vi "4461 - Create Reference Waveforms.vi"(8 "error in (no error)":errorcluster, 10 "reset signal":bool, 11 "Lockin.DAQ in":refnum<class "Lockin.DAQ.lvclass">) -> (0 "error out":errorcluster, 2 "Ref Array":waveform(dbl)[](array[waveform]), 3 "Lockin.DAQ out":refnum<class "Lockin.DAQ.lvclass">)   [LabVIEW 2016, in "Lockin.DAQ.lvclass"]
uses:
  Lockin.DAQ.lvclass
  Typedefs/REF-cluster.ctl
  Instrument.Lockinl.UI/Typedefs/REF Channel--Cluster.ctl
  Typedefs/Sampling.ctl
  <vilib>/measure/NI_MABase.lvlib
  Instrument.Lockinl.UI/Instrument.Lockin.UI.lvclass
panel:
  in  "Configuration.Channels: REF":T1 {"Order" min=1; "TC" min=0.0001 format="%#_3p"; "Phase" format="%.3g"; "Frequency" min=0.0001 max=10000.0 format="%.3g"}
  in  "Update Graph?":bool
  out "Waveform Graph":waveform(dbl)[](graph)
  out "Numeric":i32
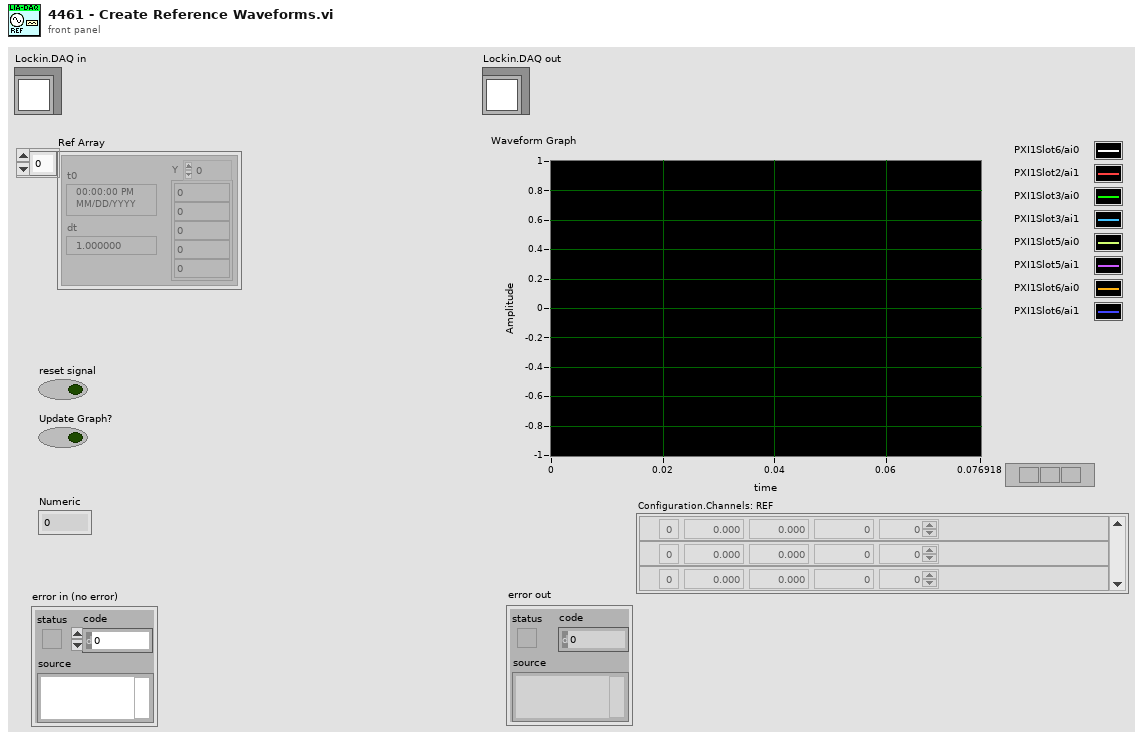
[diagram p1: front panel]
types:
  T1 = typedef "Lockin.DAQ.lvclass/REF-cluster.ctl" = T2[]
  T2 = typedef "Instrument.Lockin.UI.lvclass/REF Channel--Cluster.ctl" = cluster{"Channel":i32, "Frequency":dbl, "Phase":dbl, "TC":dbl, "Order":i32}
  T3 = typedef "Lockin.DAQ.lvclass/Sampling.ctl" = cluster{"Fs":dbl, "#s":i32}
  T4 = enum16{"Sine Wave", "Triangle Wave", "Square Wave", "Sawtooth Wave"}
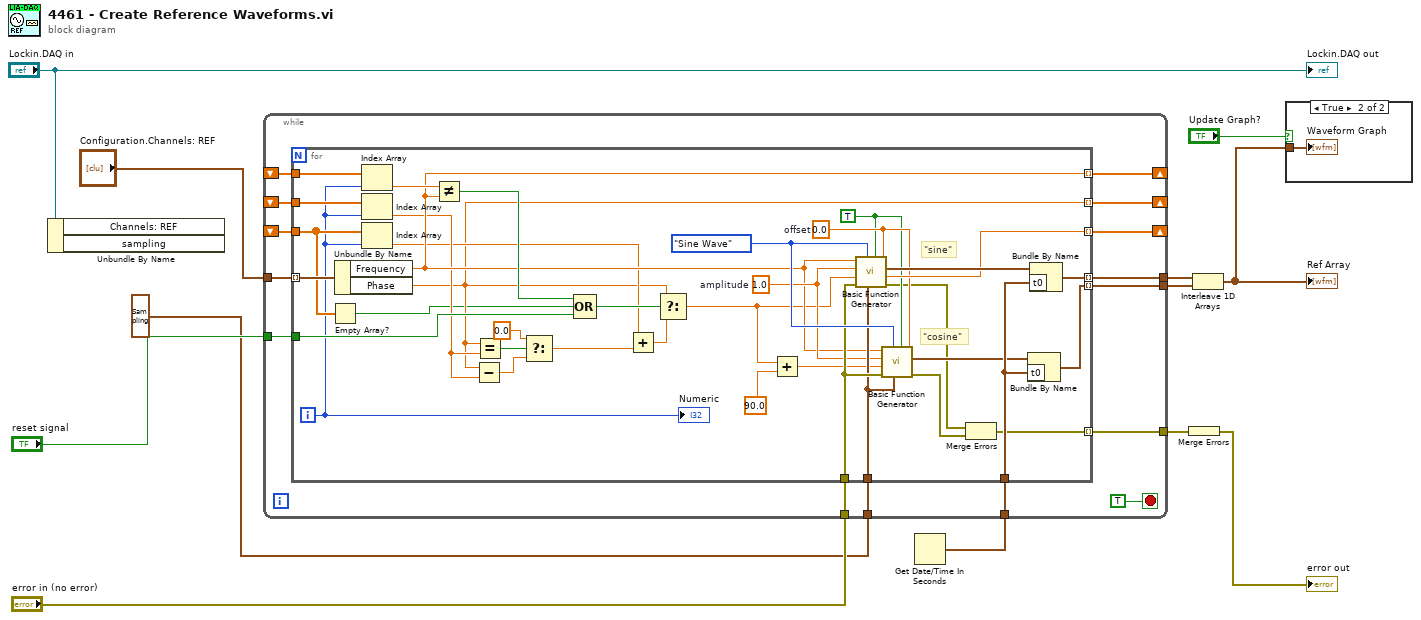
[diagram p0: block diagram]
diagram:
  n1 = Unbundle By Name("Lockin.DAQ in") -> ()  [unwired: 2 out]
  n2 = Get Date/Time In Seconds() -> (seconds since 1Jan1904=w9:timestamp)
  n3 = while {
    tunnel: T3 {"Fs"=204789.0, "#s"=15753} ("Configuration.DAQ.sampling") -> [w27]
    tunnel: [w26] -> w6
    shift-right: [w24] -> _
    shift-left: _ -> [w19]
    tunnel: w9 -> [w23]
    tunnel: "reset signal" -> [w16]
    tunnel: [w22] -> w11
    tunnel: "error in (no error)" -> [w21]
    tunnel: "Configuration.Channels: REF" -> [w20]
    shift-right: [w18] -> _
    shift-left: _ -> [w14]
    shift-right: [w17] -> _
    shift-left: _ -> [w15]
    tunnel: [w13] -> w1
    stop <- TRUE stop-if-true
    n4 = for {
      tunnel: [w63] -> w26 mode=indexing
      tunnel: w27 -> [w54]
      tunnel: [w61] -> w24 mode=indexing
      tunnel: w23 -> [w60]
      tunnel: [w58] -> w22 mode=indexing
      tunnel: w21 -> [w55]
      tunnel: w20 -> [w51] mode=indexing
      tunnel: w19 -> [w49]
      tunnel: [w42] -> w18 mode=indexing
      tunnel: [w30] -> w17 mode=indexing
      tunnel: w16 -> [w44]
      tunnel: w15 -> [w47]
      tunnel: w14 -> [w46]
      tunnel: [w33] -> w13 mode=indexing
      i -> [w43]
      w50 = TRUE ("reset signal")
      w56 = 0.0  # offset
      w57 = T4."Sine Wave" ("signal type")
      w52 = 1.0  # amplitude
      # "\"cosine\""
      # "\"sine\""
      n5 = Empty Array?(array=w49) -> (empty?=w29:bool)
      n6 = Unbundle By Name(w51) -> ("Frequency"=w42:dbl, "Phase"=w30:dbl)
      n7 = Index Array(array=w46, index=w43) -> (element=w45:dbl)
      n8 = Index Array(array=w47, index=w43) -> (element=w38:dbl)
      n9 = Index Array(array=w49, index=w43) -> (element=w31:dbl)
      n10 = Not Equal?(x=w45, y=w42) -> (x != y?=w48:bool)
      n11 = Subtract(x=w30, y=w38) -> (x-y=w41:dbl)
      n12 = Equal?(x=w30, y=w38) -> (x = y?=w40:bool)
      n13 = Select(t=0.0, s=w40, f=w41) -> (s? t:f=w32:dbl)
      n14 = Compound Arithmetic op=OR(w48, w29, w44) -> (w37:bool)
      n15 = Add(x=w31, y=w32) -> (x+y=w36:dbl)
      n16 = Select(t=w30, s=w37, f=w36) -> (s? t:f=w28:dbl)
      n17 = Add(x=w28, y=90.0) -> (x+y=w53:dbl)
      n18 = call <vilib>:"Basic Function Generator.vi"("offset"=w56, "reset signal"=w50, "sampling info"=w54, "signal type"=w57, "error in (no error)"=w55, "phase"=w28, "amplitude"=w52, "frequency"=w42) -> ("error out"=w34:errorcluster, "phase out"=w61:dbl, "signal out"=w64:waveform(dbl))  [unwired: 1 in]
      n19 = call <vilib>:"Basic Function Generator.vi"("offset"=w56, "reset signal"=w50, "sampling info"=w54, "signal type"=w57, "error in (no error)"=w55, "phase"=w53, "amplitude"=w52, "frequency"=w42) -> ("error out"=w35:errorcluster, "signal out"=w59:waveform(dbl))  [unwired: 1 in, 1 out]
      n20 = Merge Errors(w34, w35) -> (w33:errorcluster)
      n21 = Bundle By Name(cluster=w59, "t0"=w60) -> (w58:waveform(dbl))
      n22 = Bundle By Name(cluster=w64, "t0"=w60) -> (w63:waveform(dbl))
      "Numeric" <- w43
    }
  }
  n23 = Merge Errors(w1) -> (→"error out":errorcluster)
  n24 = Interleave 1D Arrays(w6, w11) -> (w7:waveform(dbl)[])
  "Ref Array" <- w7
  n25 = case shown="True" "Update Graph?" {
    tunnel: w7 -> [_ w65]
    frame False {
    }
    frame True {
      "Waveform Graph" <- w65
    }
  }
  "Lockin.DAQ out" <- "Lockin.DAQ in"
